vi "Test Static Complex Numbers 1.vi"() -> ()   [LabVIEW 2014]
uses:
  <vilib>/LabVIEW Universal Transcriptor/LabVIEW for Arduino Complex Numbers Static/ComplexNumberStatic.lvclass
panel:
  out "Error Out":errorcluster
  in  "error in":errorcluster
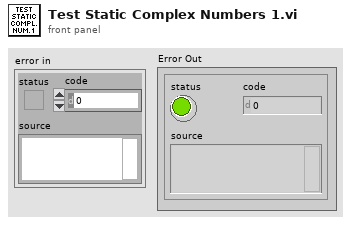
[diagram p1: front panel]
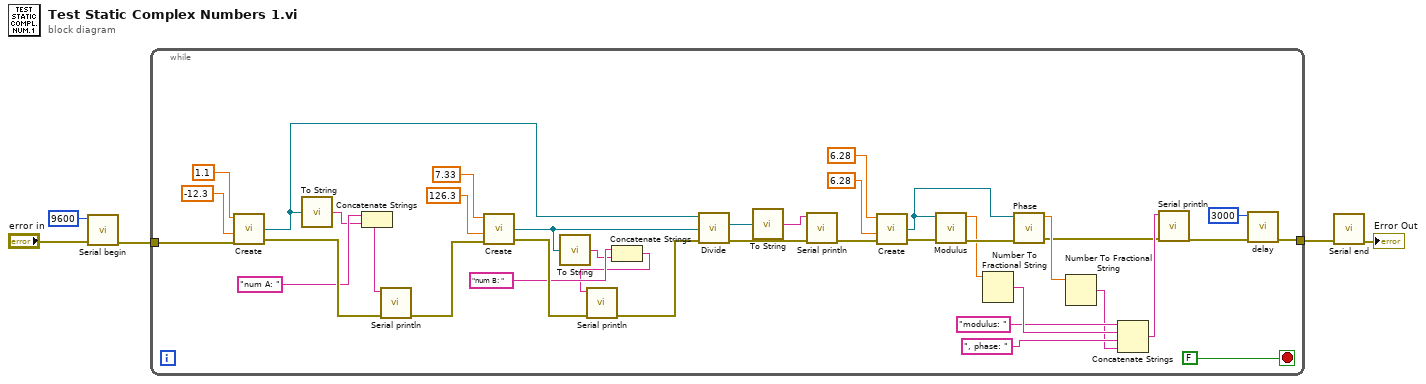
[diagram p0: block diagram]
diagram:
  n1 = call <vilib>:"Serial begin.vi"("Error In"="error in", "speed (Bd)"=9600) -> ("Error Out"=w4:errorcluster)  [unwired: 9 in]
  n2 = while {
    tunnel: w4 -> [w38]
    tunnel: [w8] -> w3
    stop <- FALSE stop-if-true
    n3 = call <vilib>:"Create.vi"("error in (no error)"=w38, "Imag"=-12.3 ("Real"), "Real"=1.1) -> ("error out"=w34:errorcluster, "ComplexNumber"=w30:refnum<class "ComplexNumberStatic.lvclass">)  [unwired: 2 in]
    n4 = call <vilib>:"To String.vi"("A"=w30) -> ("String complex num."=w26:string)
    n5 = Concatenate Strings("num A: " ("string"), w26) -> (w29:string)
    n6 = call <vilib>:"Serial println.vi"("Error In"=w34, "string in"=w29) -> ("Error Out"=w33:errorcluster)  [unwired: 9 in]
    n7 = call <vilib>:"Create.vi"("error in (no error)"=w33, "Imag"=126.3 ("Real"), "Real"=7.33) -> ("error out"=w32:errorcluster, "ComplexNumber"=w28:refnum<class "ComplexNumberStatic.lvclass">)  [unwired: 2 in]
    n8 = call <vilib>:"To String.vi"("A"=w28) -> ("String complex num."=w24:string)
    n9 = Concatenate Strings("num B: " ("string"), w24) -> (w23:string)
    n10 = call <vilib>:"Serial println.vi"("Error In"=w32, "string in"=w23) -> ("Error Out"=w31:errorcluster)  [unwired: 9 in]
    n11 = call <vilib>:"Divide.vi"("error in (no error)"=w31, "B"=w28, "A"=w30) -> ("error out"=w37:errorcluster, "A/B"=w39:refnum<class "ComplexNumberStatic.lvclass">)  [unwired: 7 in]
    n12 = call <vilib>:"To String.vi"("A"=w39) -> ("String complex num."=w36:string)
    n13 = call <vilib>:"Serial println.vi"("Error In"=w37, "string in"=w36) -> ("Error Out"=w22:errorcluster)  [unwired: 9 in]
    n14 = call <vilib>:"Create.vi"("error in (no error)"=w22, "Imag"=6.28 ("Real"), "Real"=6.28) -> ("error out"=w19:errorcluster, "ComplexNumber"=w17:refnum<class "ComplexNumberStatic.lvclass">)  [unwired: 2 in]
    n15 = call <vilib>:"Modulus.vi"("error in (no error)"=w19, "A"=w17) -> ("error out"=w18:errorcluster, "modul"=w16:dbl)  [unwired: 8 in]
    n16 = Number To Fractional String(number=w16) -> (F-format string=w14:string)  [unwired: 3 in]
    n17 = call <vilib>:"Phase.vi"("error in (no error)"=w18, "A"=w17) -> ("error out"=w9:errorcluster, "phase"=w15:dbl)  [unwired: 8 in]
    n18 = Number To Fractional String(number=w15) -> (F-format string=w11:string)  [unwired: 3 in]
    n19 = Concatenate Strings("modulus: " ("string"), w14, ", phase: " ("string"), w11) -> (w10:string)
    n20 = call <vilib>:"Serial println.vi"("Error In"=w9, "string in"=w10) -> ("Error Out"=w7:errorcluster)  [unwired: 9 in]
    n21 = call <vilib>:"delay.vi"("Error In"=w7, "time (ms)"=3000) -> ("Error Out"=w8:errorcluster)  [unwired: 9 in]
  }
  n22 = call <vilib>:"Serial end.vi"("Error In"=w3) -> ("Error Out"=→"Error Out":errorcluster)  [unwired: 10 in]
